vi "Smista AO.vi"(0 "AO scalati IN":T3, 7 "Forza AO cDAQ":T1, 9 "Forza AO plc_3":T2) -> (8 "StatoAO cDAQ out":T1, 15 "statoAO_PLC 3 out":T2)   [LabVIEW 2019]
uses:
  TypeDef/Lista AO sistema.ctl
  cDAQ_PLC Folder/controls/statoAO_plc_3.ctl
  GlobalForzaUscite.vi
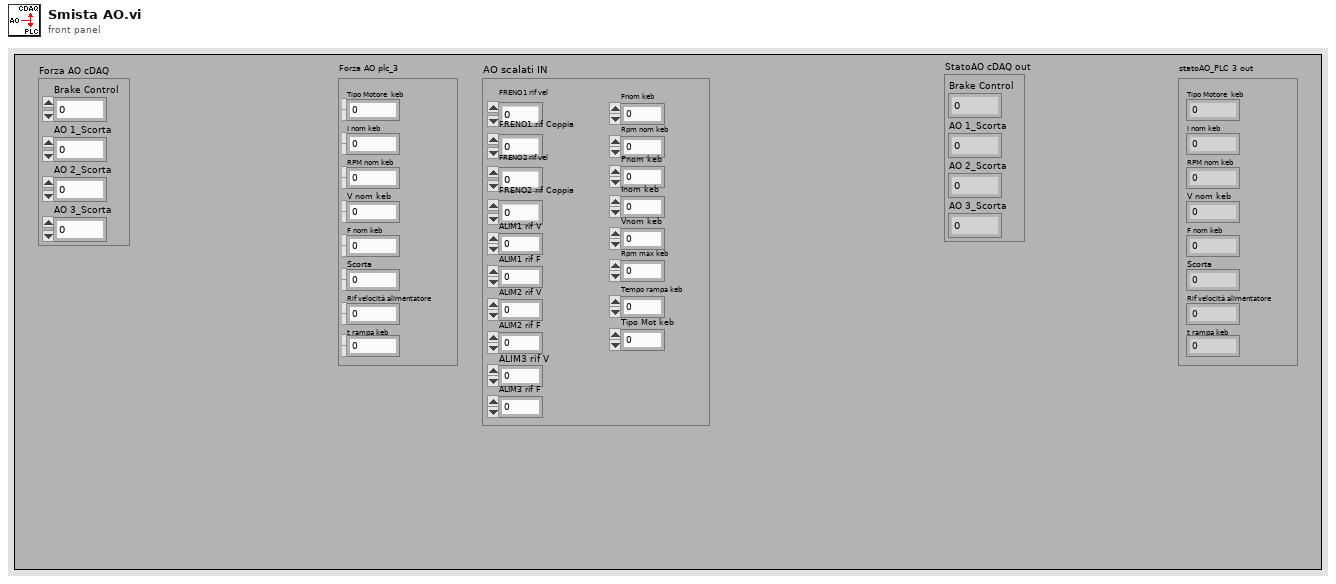
[diagram p1: front panel]
types:
  T1 = cluster{"Brake Control":dbl, "AO 1_Scorta":dbl, "AO 2_Scorta":dbl, "AO 3_Scorta":dbl}
  T2 = typedef "statoAO_plc_3.ctl" = cluster{"Tipo Motore  keb":dbl, "I nom keb":dbl, "RPM nom keb":dbl, "V nom keb":dbl, "F nom keb":dbl, "Scorta":dbl, "Rif velocità alimentatore":dbl, "t rampa keb":dbl}
  T3 = typedef "Lista AO sistema.ctl" = cluster{"FRENO1 rif vel":dbl, "FRENO1 rif Coppia":dbl, "FRENO2 rif vel":dbl, "FRENO2 rif Coppia":dbl, "ALIM1 rif V":dbl, "ALIM1 rif F":dbl, "ALIM2 rif V":dbl, "ALIM2 rif F":dbl, "ALIM3 rif V":dbl, "ALIM3 rif F":dbl, "Fnom keb":dbl, "Rpm nom keb":dbl, "Pnom keb":dbl, "Inom keb":dbl, "Vnom keb":dbl, "Rpm max keb":dbl, "Tempo rampa keb":dbl, "Tipo Mot keb":dbl}
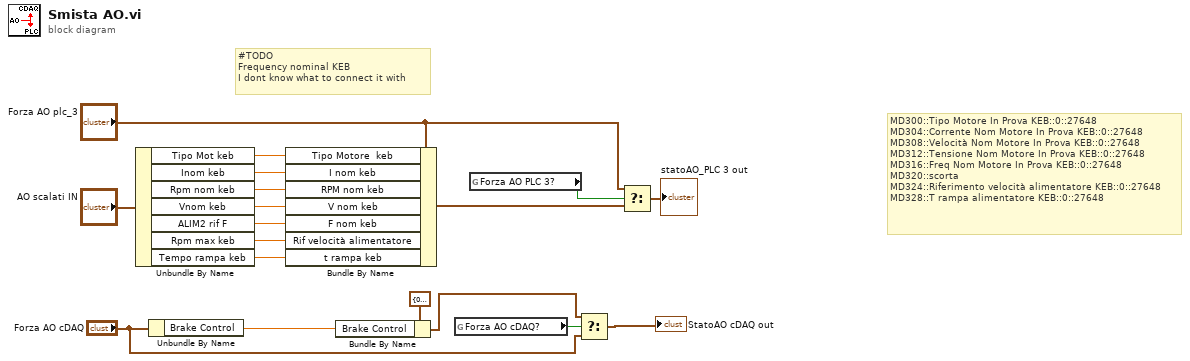
[diagram p0: block diagram]
diagram:
  # "#TODO\nFrequency nominal KEB \nI dont know what to connect it with"
  # "MD300::Tipo Motore In Prova KEB::0::27648\nMD304::Corrente Nom Motore In Prova KEB::0::27648\nMD308::Velocità Nom Motore In Prova KEB::0::27648\nMD312::Tensione Nom Motore In Prova KEB::0::27648\nMD316::Freq Nom Motore In Prova KEB::0::27648\nMD320::scorta\nMD324::Riferimento velocità alimentatore KEB::0::27648\nMD328::T rampa alimentatore KEB::0::27648"
  n1 = Unbundle By Name("AO scalati IN") -> ("Tipo Mot keb"=w8:dbl, "Inom keb"=w7:dbl, "Rpm nom keb"=w6:dbl, "Vnom keb"=w5:dbl, "ALIM2 rif F"=w2:dbl, "Rpm max keb"=w3:dbl, "Tempo rampa keb"=w4:dbl)
  n2 = Unbundle By Name("Forza AO cDAQ") -> ("Brake Control"=w13:dbl)
  n3 = Bundle By Name(cluster="Forza AO plc_3", "Tipo Motore  keb"=w8, "I nom keb"=w7, "RPM nom keb"=w6, "V nom keb"=w5, "F nom keb"=w2, "Rif velocità alimentatore"=w3, "t rampa keb"=w4) -> (w1:T2)
  n4 = Bundle By Name(cluster=T1 {"Brake Control"=0.0, "AO 1_Scorta"=0.0, "AO 2_Scorta"=0.0, "AO 3_Scorta"=0.0} ("Mod 5_WRITE"), "Brake Control"=w13) -> (w11:T1)
  n5 = global read "GlobalForzaUscite.vi" "Forza AO cDAQ?"() -> (w17:bool)
  n6 = global read "GlobalForzaUscite.vi" "Forza AO PLC 3?"() -> (w16:bool)
  n7 = Select(t=w11, s=w17, f="Forza AO cDAQ") -> (s? t:f=→"StatoAO cDAQ out":T1)
  n8 = Select(t="Forza AO plc_3", s=w16, f=w1) -> (s? t:f=→"statoAO_PLC 3 out":T2)
